vi "Configure.vi"(8 "error in (no error)":errorcluster, 11 "Waveform in":refnum<class "Waveform.lvclass">) -> (0 "error out":errorcluster, 2 "cancelled?":bool, 3 "Waveform out":refnum<class "Waveform.lvclass">)   [LabVIEW 2012, in "Waveform.lvclass"]
doc: "The configure method configures the details for the RabbitMQ connection, the observers and the mapping script.\n\nIn the derived class, make a call to the parent for setting these parameters."
uses:
  Waveform.lvclass
  <vilib>/Utility/miscctls.llb/LVPointTypeDef.ctl
  Waveform.lvclass/Waveform.ctl
  <vilib>/Distrio/Murmex/Murmex/Murmex.lvclass
panel:
  in  "button::cancel":bool
  in  "button::ok":bool
  in  "button::configure murmex":bool
  in  "Tab Control":T1(tab)
  in  "Output Terminal C1":tag="/Dev1/PFI12" caption="Output Terminal"
  in  "C1":tag="Dev1/ctr0" caption="Counter"
  in  "PI stage trigger":tag
  in  "% camera frame rate":dbl
  in  "Duty cycle":dbl
  in  "AO clock source":tag
  in  "Galvo Physical Channels":tag="Dev1/ao0" caption="Physical Channel"
  in  "min Voltage":dbl
  in  "max Voltage":dbl
  in  "Shutter line":tag="Dev1/port0/line0:7"
  in  "Tomo":string
  in  "Stack":string
  in  "target component ID":string
  in  "AddRelayTarget":bool
  in  "RemoveRelayTarget":bool
  in  "relay start/stop to...":i32(listbox)
  in  "Orca- Master":string
  # "RabbitMQ parameters"
  # "Window position"
  # "Sends a setting or configuration value to an observer, e.g. observer.parameter=settingsname;"
  # "Frame trigger"
  # "Galvo"
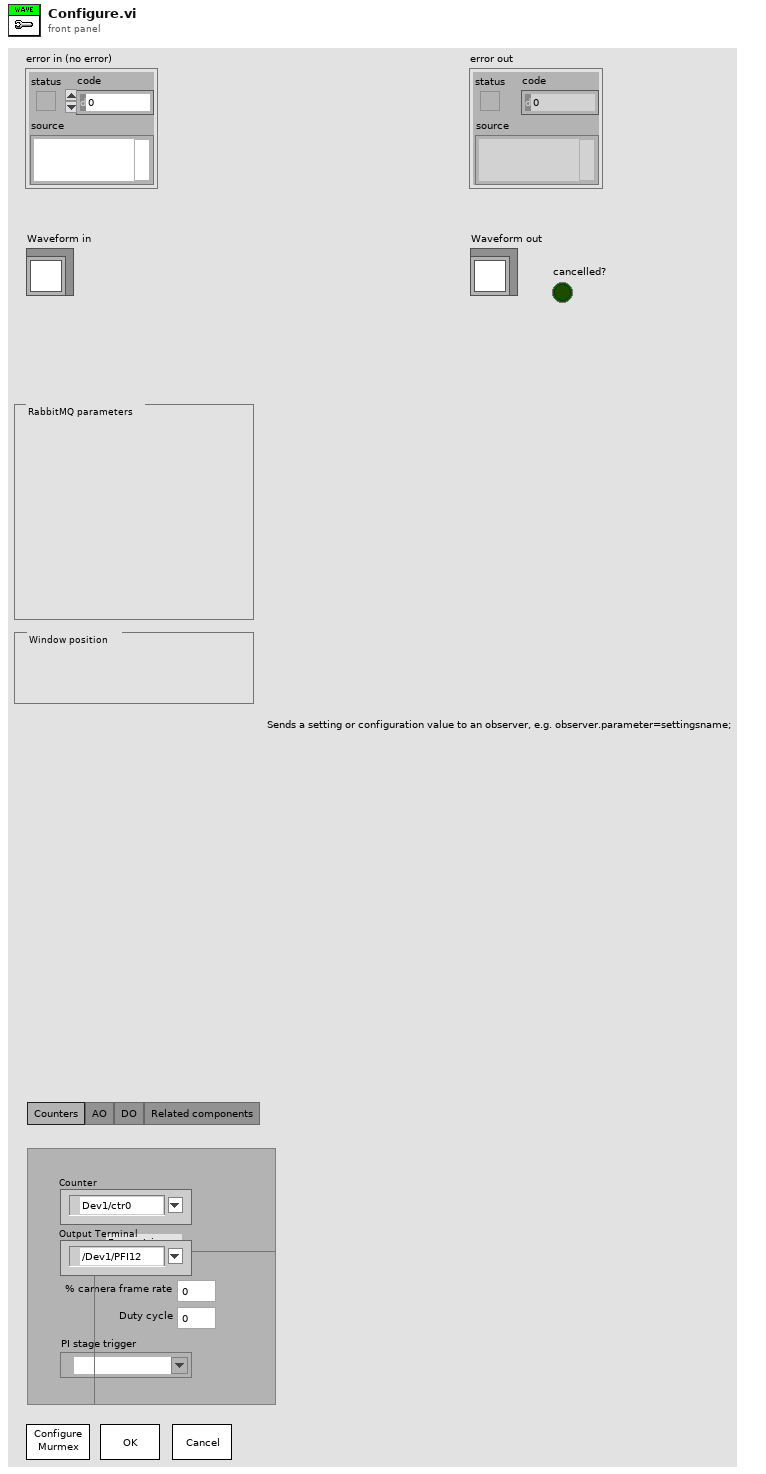
[diagram p1: front panel]
types:
  T1 = enum32{"Counters", "AO", "DO", "Related components"}
  T2 = typedef "LVPointTypeDef.ctl" = cluster{"Horizontal":i16, "Vertical":i16}
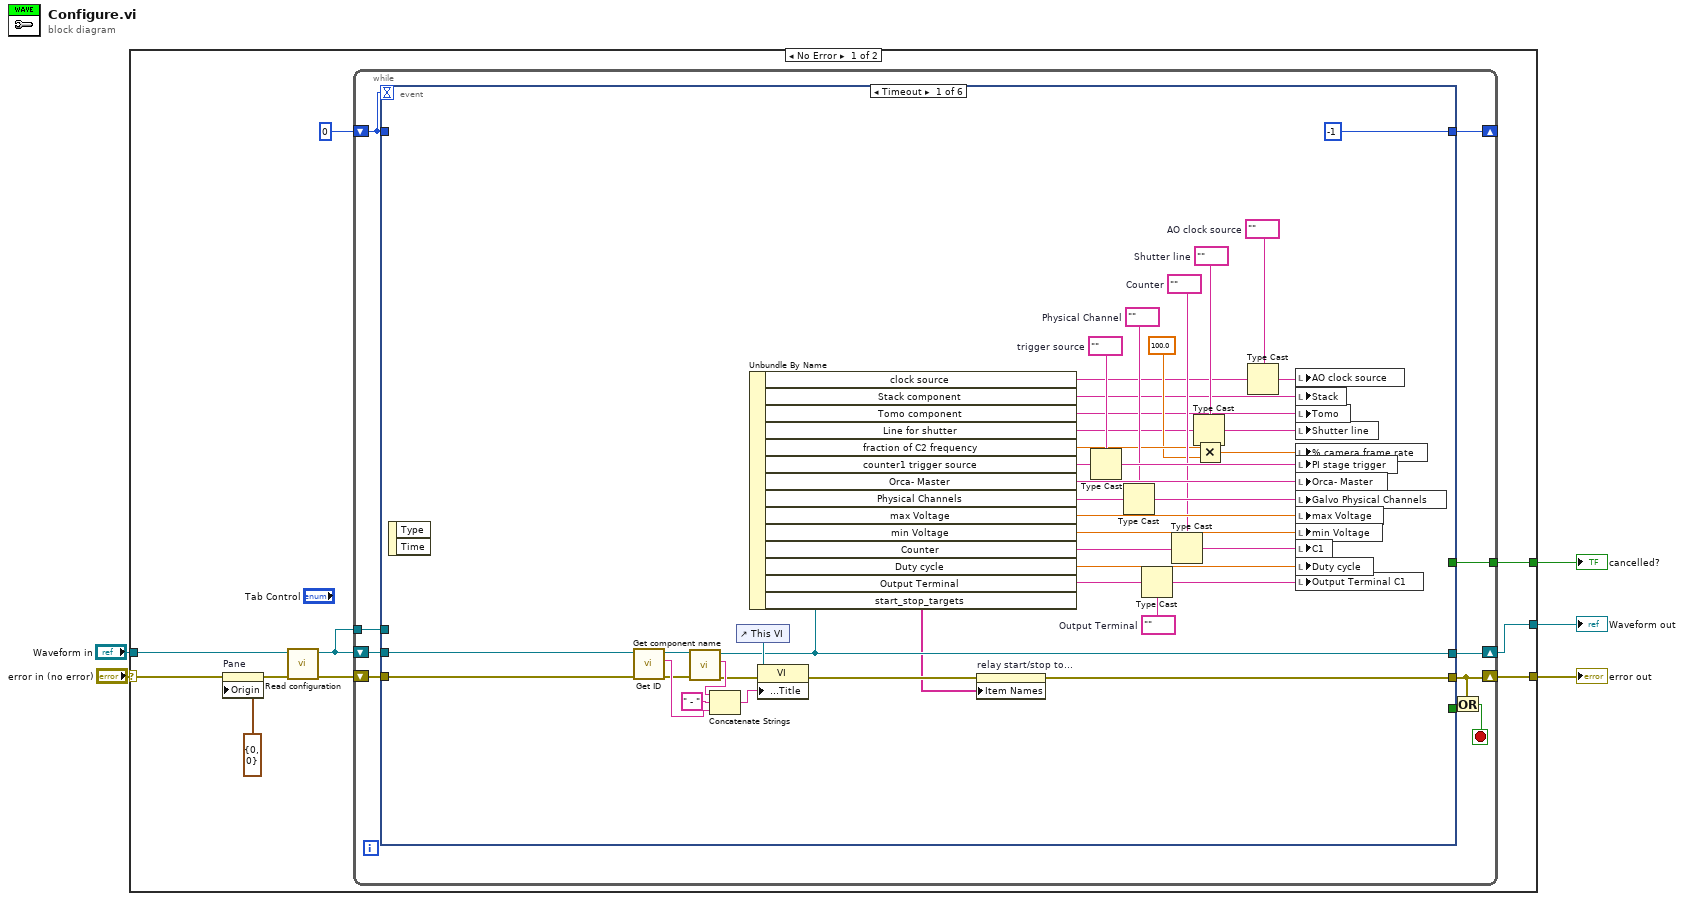
[diagram p0: block diagram]
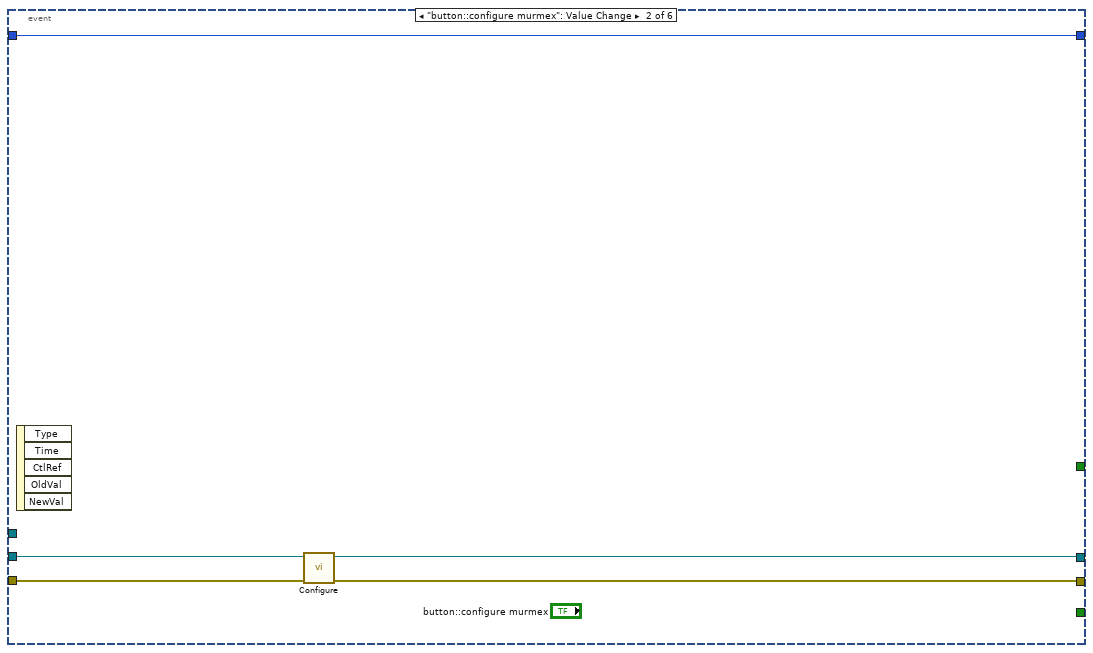
[diagram p2: hidden frame]
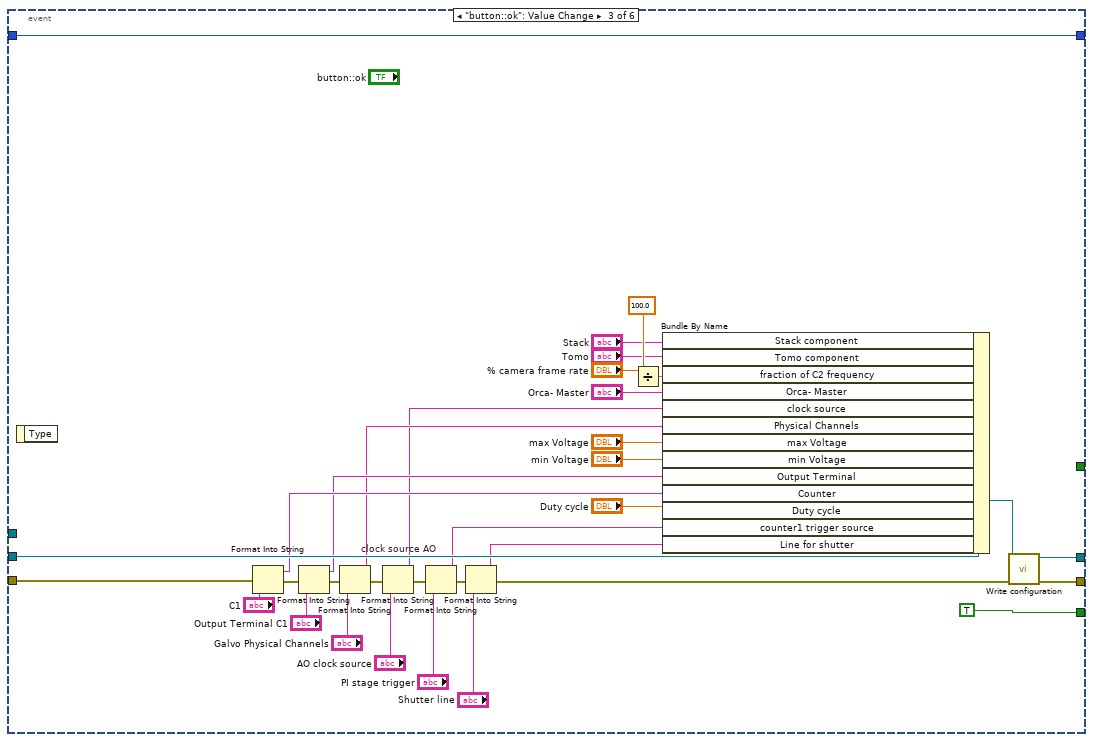
[diagram p3: hidden frame]
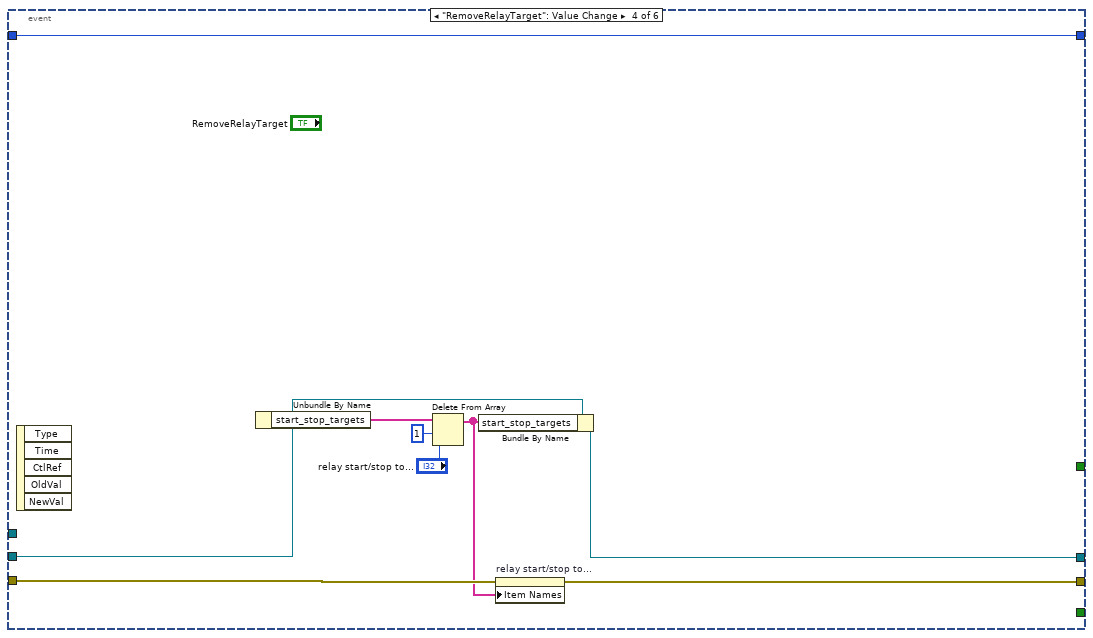
[diagram p4: hidden frame]
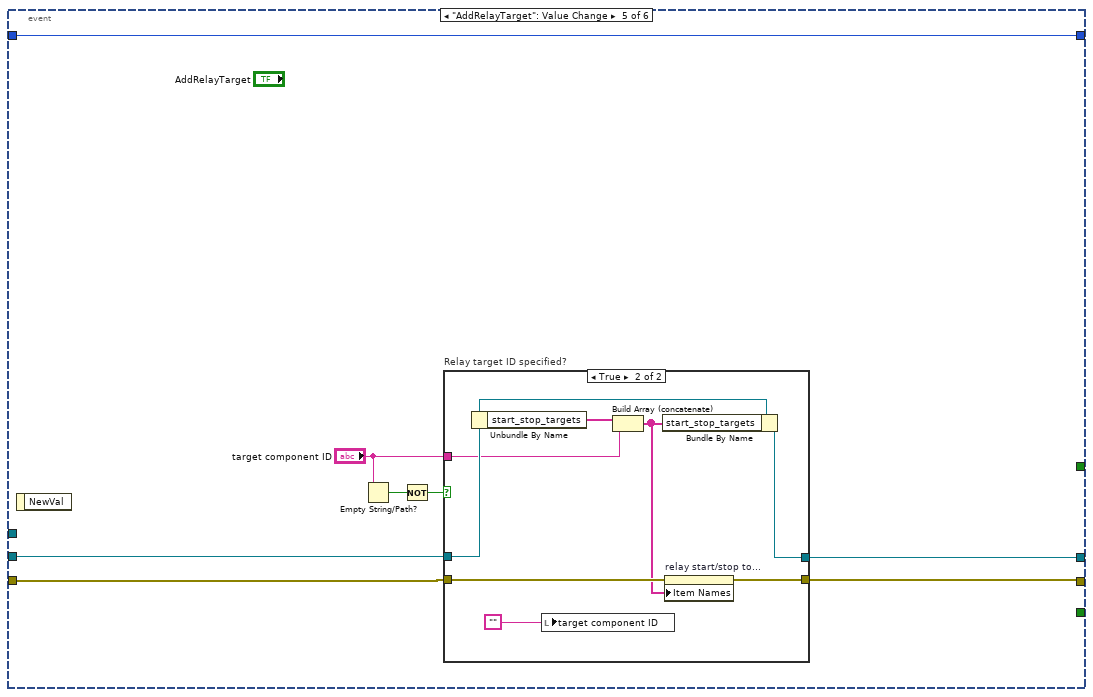
[diagram p5: hidden frame]
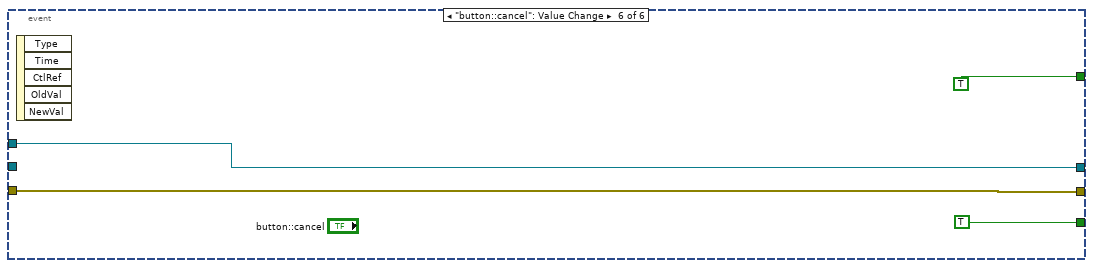
[diagram p7: hidden frame]
diagram:
  n1 = case shown="No Error" "error in (no error)" {
    selector: "error in (no error)" -> [w14 w139]
    tunnel: "Waveform in" -> [w12 w138]
    tunnel: [w8 w139] -> w3
    tunnel: [w7 w138] -> w2
    tunnel: [w6 _] -> w1
    frame No Error {
      n2 = property on="Pane" class="Pane"(error in=w14, "Origin"=T2 {"Horizontal"=0, "Vertical"=0}) -> (error out=w13:errorcluster)  [unwired: 1 in, 1 out]
      n3 = call <vilib>:"Read configuration.vi"("error in (no error)"=w13, "Murmex in"=w12) -> ("error out"=w11:errorcluster, "Murmex out"=w10:refnum<class "Waveform.lvclass">)  [unwired: 7 in, 1 out]
      n4 = while {
        shift-right: [w19] -> w8
        shift-left: w11 -> [w25]
        shift-right: [w21] -> w7
        shift-left: w10 -> [w23]
        tunnel: w10 -> [w24]
        shift-right: [w20] -> _
        shift-left: 0 -> [w22]
        tunnel: [w16] -> w6
        stop <- w18 stop-if-true
        n5 = event shown="[0] Timeout" {
          selector: _ -> [_ _ _ _ _ _]
          dyn-events: _ -> [_ _ _ _ _ _]
          timeout: w22 -> [_ _ _ _ _ _]
          tunnel: w25 -> [w67 w72 w97 w109 w119 w137]
          tunnel: w24 -> [_ _ _ _ _ w136]
          tunnel: w23 -> [w66 w69 w98 w111 w122 _]
          tunnel: w22 -> [_ w70 w99 w115 w123 _]
          tunnel: [w38 w71 w105 w108 w118 w137] -> w19
          tunnel: [w57 w68 w106 w110 w121 w136] -> w21
          tunnel: [-1 w70 w99 w115 w123 _] -> w20
          tunnel: [_ _ TRUE _ _ TRUE ("force loading?")] -> w17
          tunnel: [_ _ _ _ _ TRUE ("force loading?")] -> w16
          event Timeout {
            w28 = tag ""  # AO clock source
            w31 = tag ""  # Shutter line
            w40 = tag ""  # Counter
            w42 = tag ""  # trigger source
            w45 = tag ""  # Output Terminal
            w41 = tag ""  # Physical Channel
            n6 = event-data() -> ()  [unwired: 1 in, 2 out]
            n7 = call <vilib>:"Get ID.vi"("error in (no error)"=w67, "Murmex in"=w66) -> ("error out"=w61:errorcluster, "component id"=w64:string, "Murmex out"=w62:refnum<class "Waveform.lvclass">)  [unwired: 7 in]
            n8 = call <vilib>:"Get component name.vi"("error in (no error)"=w61, "Murmex in"=w62) -> ("error out"=w59:errorcluster, "component name"=w63:string, "Murmex out"=w57:refnum<class "Waveform.lvclass">)  [unwired: 7 in]
            n9 = Concatenate Strings(w63, " - " ("string"), w64) -> (w58:string)
            n10 = control-ref of="This VI"() -> (w60:refnum<vi>)
            n11 = Unbundle By Name(w57) -> ("clock source"=w26:string, "Stack component"=w29:string, "Tomo component"=w30:string, "Line for shutter"=w33:string, "fraction of C2 frequency"=w36:dbl, "counter1 trigger source"=w44:string, "Orca- Master"=w52:string, "Physical Channels"=w50:string, "max Voltage"=w53:dbl, "min Voltage"=w54:dbl, "Counter"=w48:string, "Duty cycle"=w55:dbl, "Output Terminal"=w46:string, "start_stop_targets"=w37:string[])
            n12 = property class="VI"(reference=w60, error in=w59, "Front Panel.Title"=w58) -> (error out=w39:errorcluster)  [unwired: 1 out]
            n13 = property on="relay start/stop to..." class="LstBox (strict)"(error in=w39, "Item Names"=w37) -> (error out=w38:errorcluster)  [unwired: 1 in, 1 out]
            n14 = Type Cast(type=w42, x=w44) -> (*(type *) &x=w43:tag)
            n15 = Type Cast(type=w41, x=w50) -> (*(type *) &x=w51:tag)
            n16 = Type Cast(type=w45, x=w46) -> (*(type *) &x=w47:tag)
            n17 = Type Cast(type=w40, x=w48) -> (*(type *) &x=w49:tag)
            n18 = Type Cast(type=w31, x=w33) -> (*(type *) &x=w32:tag)
            n19 = Multiply(x=w36, y=100.0) -> (x*y=w35:dbl)
            n20 = Type Cast(type=w28, x=w26) -> (*(type *) &x=w27:tag)
            n21 = local write "AO clock source"(w27) -> ()
            n22 = local write "Stack"(w29) -> ()
            n23 = local write "Tomo"(w30) -> ()
            n24 = local write "Shutter line"(w32) -> ()
            n25 = local write "% camera frame rate"(w35) -> ()
            n26 = local write "PI stage trigger"(w43) -> ()
            n27 = local write "Orca- Master"(w52) -> ()
            n28 = local write "Galvo Physical Channels"(w51) -> ()
            n29 = local write "max Voltage"(w53) -> ()
            n30 = local write "min Voltage"(w54) -> ()
            n31 = local write "C1"(w49) -> ()
            n32 = local write "Duty cycle"(w55) -> ()
            n33 = local write "Output Terminal C1"(w47) -> ()
          }
          event "button::configure murmex": Value Change {
            n34 = event-data() -> ()  [unwired: 1 in, 5 out]
            n35 = call-parent "Configure.vi"("error in (no error)"=w72, "Murmex in"=w69) -> ("error out"=w71:errorcluster, "Murmex out"=w68:refnum<class "Waveform.lvclass">)  [unwired: 7 in, 1 out]
          }
          event "button::ok": Value Change {
            n36 = event-data() -> ()  [unwired: 1 in, 1 out]
            n37 = Format Into String(error in=w97, "C1") -> (resulting string=w91:string, error out=w95:errorcluster)  [unwired: 2 in]
            n38 = Format Into String(error in=w95, "Output Terminal C1") -> (resulting string=w90:string, error out=w73:errorcluster)  [unwired: 2 in]
            n39 = Format Into String(error in=w73, "Galvo Physical Channels") -> (resulting string=w89:string, error out=w92:errorcluster)  [unwired: 2 in]
            n40 = Format Into String "clock source AO"(error in=w92, "AO clock source") -> (resulting string=w88:string, error out=w76:errorcluster)  [unwired: 2 in]
            n41 = Format Into String(error in=w76, "PI stage trigger") -> (resulting string=w85:string, error out=w81:errorcluster)  [unwired: 2 in]
            n42 = Format Into String(error in=w81, "Shutter line") -> (resulting string=w74:string, error out=w80:errorcluster)  [unwired: 2 in]
            n43 = Divide(x="% camera frame rate", y=100.0) -> (x/y=w82:dbl)
            n44 = Bundle By Name(cluster=w98, "Stack component"="Stack", "Tomo component"="Tomo", "fraction of C2 frequency"=w82, "Orca- Master"="Orca- Master", "clock source"=w88, "Physical Channels"=w89, "max Voltage"="max Voltage", "min Voltage"="min Voltage", "Output Terminal"=w90, "Counter"=w91, "Duty cycle"="Duty cycle", "counter1 trigger source"=w85, "Line for shutter"=w74) -> (w104:refnum<class "Waveform.lvclass">)
            n45 = call <vilib>:"Write configuration.vi"("error in (no error)"=w80, "Murmex in"=w104) -> ("error out"=w105:errorcluster, "Murmex out"=w106:refnum<class "Waveform.lvclass">)  [unwired: 8 in]
          }
          event "RemoveRelayTarget": Value Change {
            n46 = event-data() -> ()  [unwired: 1 in, 5 out]
            n47 = Unbundle By Name(w111) -> ("start_stop_targets"=w114:string[])
            n48 = Delete From Array(array=w114, length=1, index="relay start/stop to...") -> (array with subset deleted=w107:string[])  [unwired: 1 out]
            n49 = Bundle By Name(cluster=w111, "start_stop_targets"=w107) -> (w110:refnum<class "Waveform.lvclass">)
            n50 = property on="relay start/stop to..." class="LstBox (strict)"(error in=w109, "Item Names"=w107) -> (error out=w108:errorcluster)  [unwired: 1 in, 1 out]
          }
          event "AddRelayTarget": Value Change {
            n51 = event-data() -> ()  [unwired: 1 in, 1 out]
            n52 = Empty String/Path?(string/path="target component ID") -> (empty?=w117:bool)
            n53 = Not(x=w117) -> (.not. x?=w116:bool)
            n54 = case "Relay target ID specified?" shown="True" w116 {
              tunnel: w122 -> [w125 w133]
              tunnel: [w125 w132] -> w121
              tunnel: "target component ID" -> [_ w130]
              tunnel: w119 -> [w124 w128]
              tunnel: [w124 w127] -> w118
              frame False {
              }
              frame True {
                n55 = Unbundle By Name(w133) -> ("start_stop_targets"=w131:string[])
                n56 = local write "target component ID"("") -> ()
                n57 = Build Array (concatenate)(w131, w130) -> (w126:string[])
                n58 = Bundle By Name(cluster=w133, "start_stop_targets"=w126) -> (w132:refnum<class "Waveform.lvclass">)
                n59 = property on="relay start/stop to..." class="LstBox (strict)"(error in=w128, "Item Names"=w126) -> (error out=w127:errorcluster)  [unwired: 1 in, 1 out]
              }
            }
          }
          event "button::cancel": Value Change {
            n60 = event-data() -> ()  [unwired: 1 in, 5 out]
          }
        }
        n61 = Or(x=w19, y=w17) -> (x .or. y?=w18:bool)
      }
    }
    frame Error {
    }
  }
  "error out" <- w3
  "Waveform out" <- w2
  "cancelled?" <- w1
